vi "Untitled 3.vi"() -> ()   [LabVIEW 2020]
panel:
  out "agotado 3":string="Articulo agotado"
  in  "# dulce":dbl
  in  "#bebida fria":dbl
  in  "#cafe":dbl
  in  "# snack":dbl
  in  "stop":bool
  in  "Tab Control":enum32{"Page 1", "Page 2"}(tab)
  out "producto":bool
  out "cambio":bool
  in  "dulce":bool
  in  "bebida fria":bool
  in  "cafe":bool
  in  "snack":bool
  in  "Cancelar":bool
  in  "comprar":bool
  in  "Monedas":cluster{"moneda 10":bool, "moneda 20":bool}
  out "Cambio":dbl
  out "Dinero ingresado":dbl
  out "agotado":string="Articulo agotado"
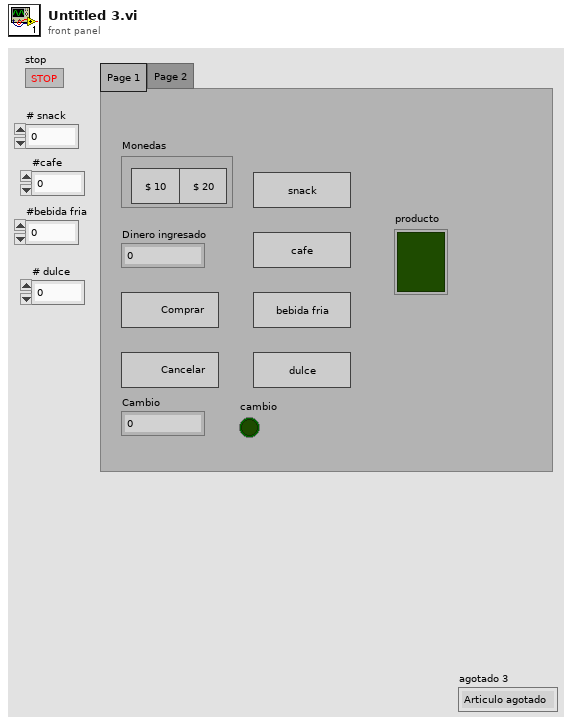
[diagram p1: front panel]
types:
  T1 = enum16{"inicio", "snack", "comprar s", "cambio s", "cafe", "comprar c", "cambio c", "bebida fria", "comprar bf", "cambio bf", "dulce", "comprar d", "cambio d", "reinicio", "cancelar"}
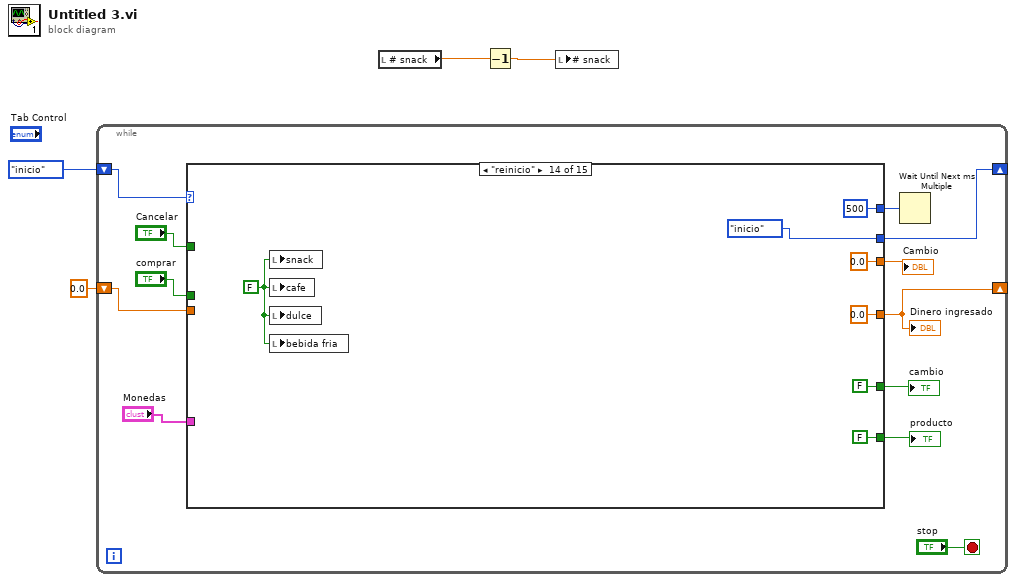
[diagram p0: block diagram]
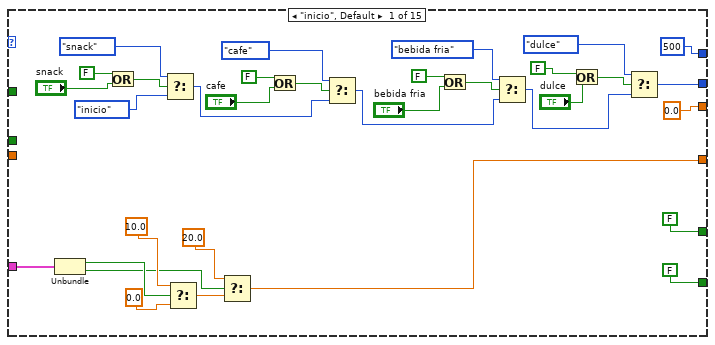
[diagram p2: hidden frame]
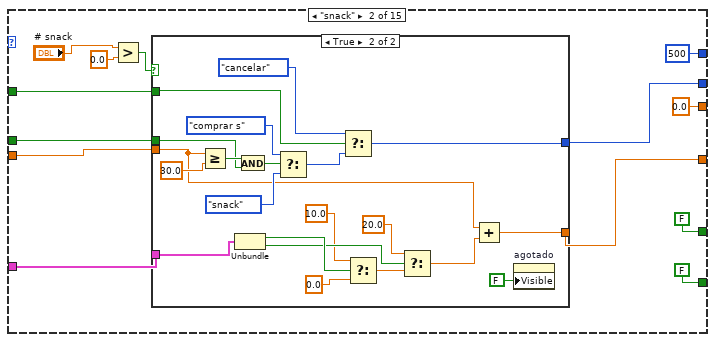
[diagram p3: hidden frame]
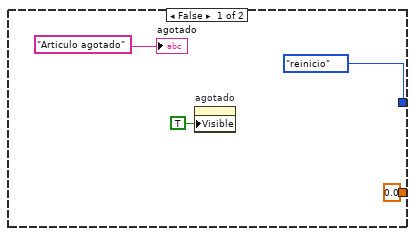
[diagram p4: hidden frame]
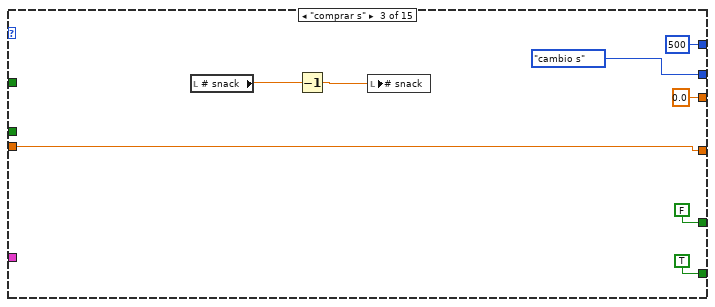
[diagram p5: hidden frame]
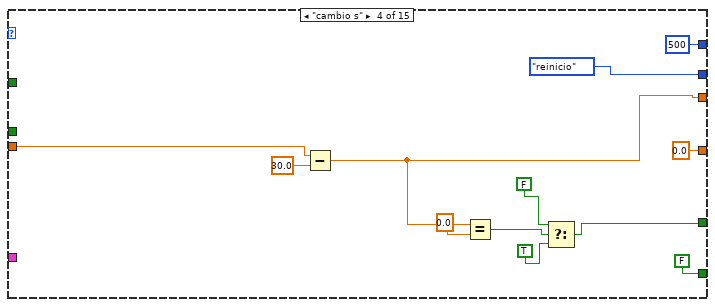
[diagram p6: hidden frame]
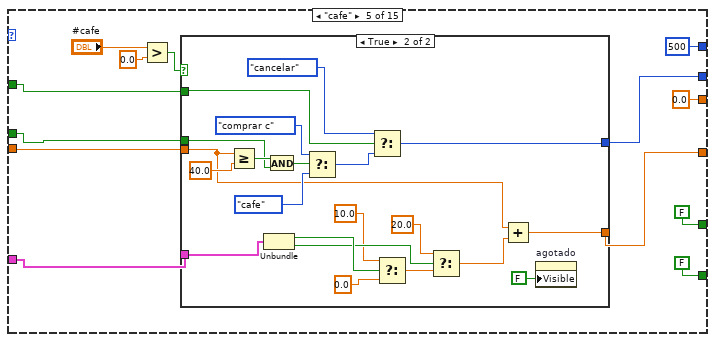
[diagram p7: hidden frame]
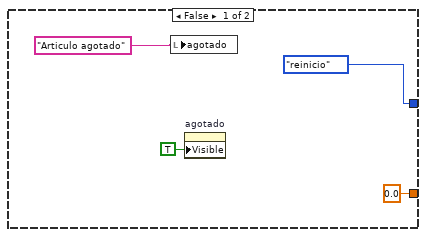
[diagram p8: hidden frame]
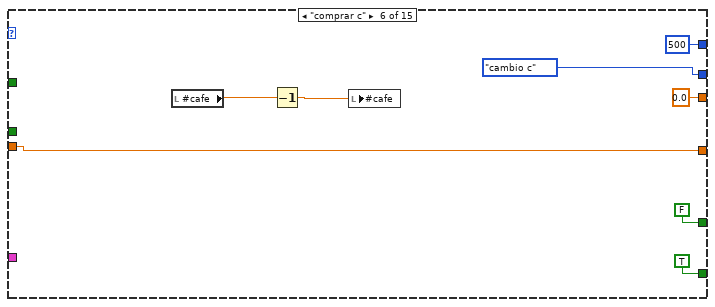
[diagram p9: hidden frame]
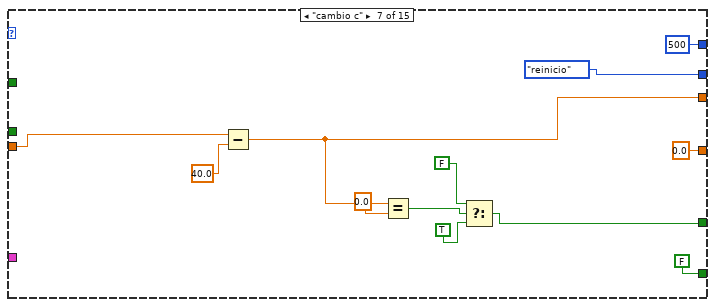
[diagram p10: hidden frame]
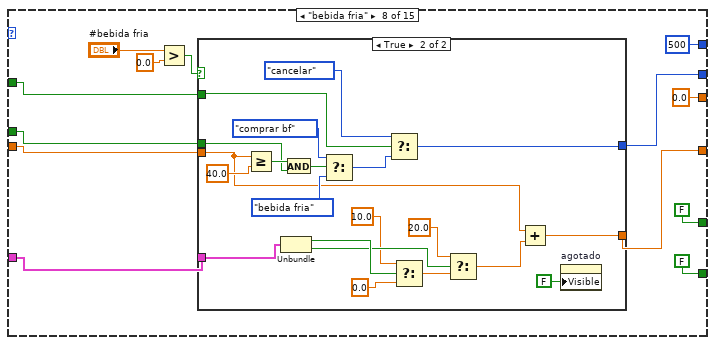
[diagram p11: hidden frame]
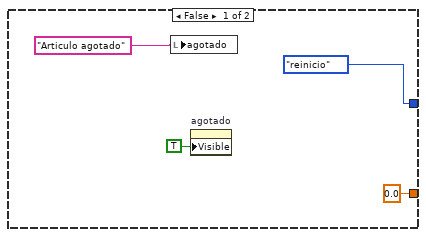
[diagram p12: hidden frame]
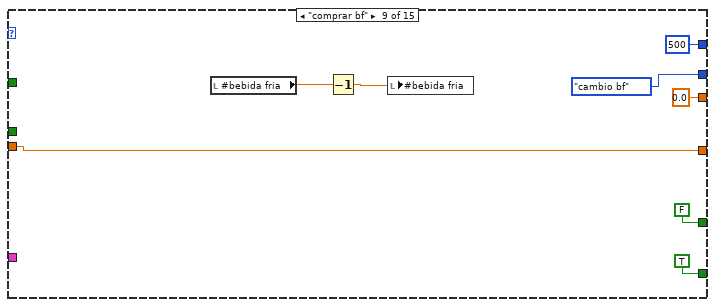
[diagram p13: hidden frame]
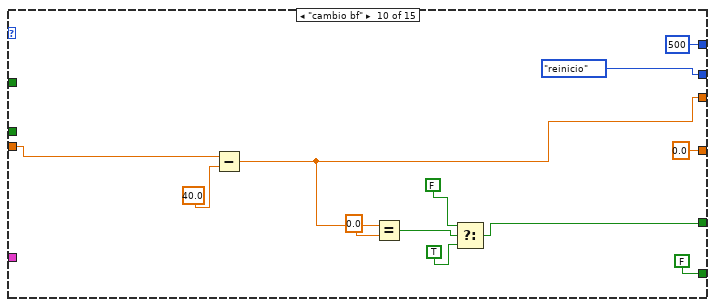
[diagram p14: hidden frame]
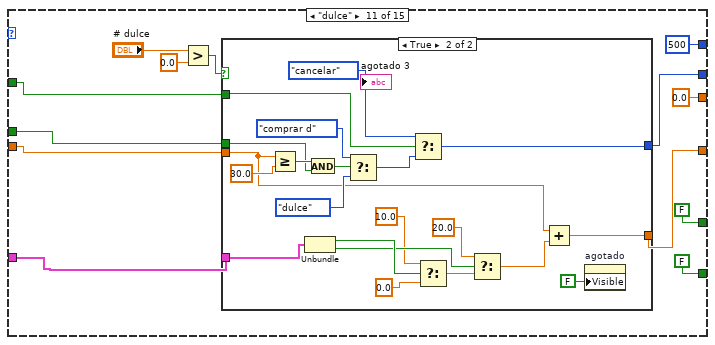
[diagram p15: hidden frame]
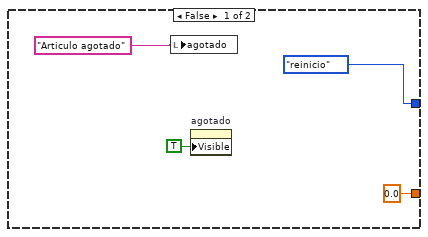
[diagram p16: hidden frame]
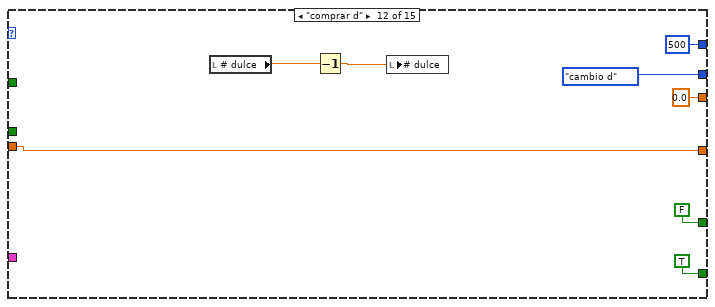
[diagram p17: hidden frame]
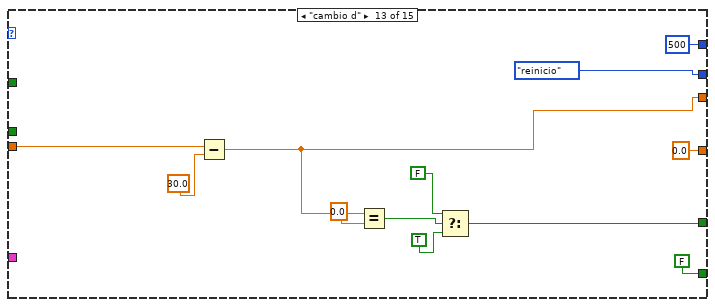
[diagram p18: hidden frame]
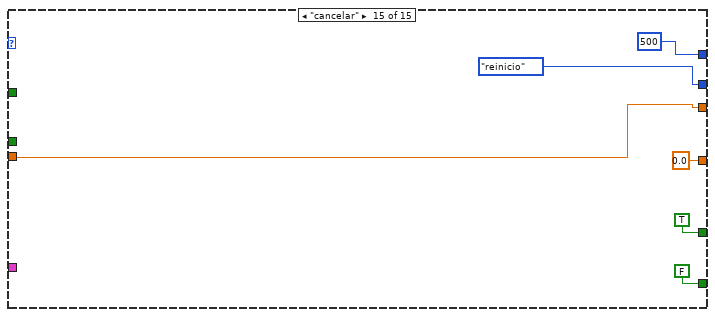
[diagram p19: hidden frame]
diagram:
  n1 = while {
    shift-right: [w14] -> _
    shift-left: T1."inicio" -> [w16]
    shift-right: [w8] -> _
    shift-left: 0.0 ("f") -> [w7]
    stop <- "stop" stop-if-true
    n2 = case shown="\"reinicio\"" w16 {
      tunnel: [500 500 500 500 500 500 500 500 500 500 500 500 500 500 500] -> w15
      tunnel: [w28 w55 T1."cambio s" T1."reinicio" w113 T1."cambio c" T1."reinicio" w171 T1."cambio bf" T1."reinicio" w228 T1."cambio d" T1."reinicio" T1."inicio" T1."reinicio"] -> w14
      tunnel: [0.0 0.0 0.0 w104 0.0 0.0 w156 0.0 0.0 w216 0.0 0.0 w273 0.0 w292] -> w13
      tunnel: "Monedas" -> [w26 w57 _ _ w114 _ _ w172 _ _ w233 _ _ _ _]
      tunnel: [w19 w56 w92 0.0 ("f") w112 w153 0.0 ("f") w168 w208 0.0 ("f") w227 w266 0.0 ("f") 0.0 ("f") 0.0 ("f")] -> w8
      tunnel: [FALSE FALSE TRUE FALSE FALSE TRUE FALSE FALSE TRUE FALSE FALSE TRUE FALSE FALSE FALSE] -> w11
      tunnel: [FALSE FALSE FALSE w100 FALSE FALSE w158 FALSE FALSE w214 FALSE FALSE w272 FALSE TRUE] -> w10
      tunnel: w7 -> [_ w60 w92 w107 w115 w153 w154 w173 w208 w212 w232 w266 w270 _ w292]
      tunnel: "comprar" -> [_ w59 _ _ w116 _ _ w174 _ _ w231 _ _ _ _]
      tunnel: "Cancelar" -> [_ w58 _ _ w117 _ _ w175 _ _ w230 _ _ _ _]
      frame "inicio", Default {
        n3 = Unbundle(w26) -> ("moneda 10"=w25:bool, "moneda 20"=w21:bool)
        n4 = Or(x=FALSE, y="snack") -> (x .or. y?=w47:bool)
        n5 = Select(t=T1."snack", s=w47, f=T1."inicio") -> (s? t:f=w40:T1)
        n6 = Select(t=10.0, s=w25, f=0.0) -> (s? t:f=w22:dbl)
        n7 = Select(t=20.0, s=w21, f=w22) -> (s? t:f=w19:dbl)
        n8 = Or(x=FALSE, y="cafe") -> (x .or. y?=w43:bool)
        n9 = Select(t=T1."cafe", s=w43, f=w40) -> (s? t:f=w35:T1)
        n10 = Or(x=FALSE, y="bebida fria") -> (x .or. y?=w38:bool)
        n11 = Select(t=T1."bebida fria", s=w38, f=w35) -> (s? t:f=w30:T1)
        n12 = Or(x=FALSE, y="dulce") -> (x .or. y?=w33:bool)
        n13 = Select(t=T1."dulce", s=w33, f=w30) -> (s? t:f=w28:T1)
      }
      frame "snack" {
        n14 = Greater?(x="# snack", y=0.0) -> (0:w61:bool)
        n15 = case shown="True" w61 {
          tunnel: w60 -> [_ w71]
          tunnel: w59 -> [_ w82]
          tunnel: w58 -> [_ w69]
          tunnel: w57 -> [_ w73]
          tunnel: [0.0 w70] -> w56
          tunnel: [T1."reinicio" w68] -> w55
          frame False {
            n16 = property on="agotado" class="Str"("Visible"=TRUE) -> ()  [unwired: 2 in, 2 out]
            "agotado" <- "Articulo agotado"
          }
          frame True {
            n17 = Greater Or Equal?(x=w71, y=30.0) -> (x >= y?=w86:bool)
            n18 = Unbundle(w73) -> ("moneda 10"=w79:bool, "moneda 20"=w77:bool)
            n19 = And(x=w86, y=w82) -> (x .and. y?=w87:bool)
            n20 = Select(t=T1."comprar s", s=w87, f=T1."snack") -> (s? t:f=w81:T1)
            n21 = Select(t=T1."cancelar", s=w69, f=w81) -> (s? t:f=w68:T1)
            n22 = Select(t=10.0, s=w79, f=0.0) -> (s? t:f=w78:dbl)
            n23 = Select(t=20.0, s=w77, f=w78) -> (s? t:f=w72:dbl)
            n24 = Add(x=w71, y=w72) -> (x+y=w70:dbl)
            n25 = property on="agotado" class="Str"("Visible"=FALSE) -> ()  [unwired: 2 in, 2 out]
          }
        }
      }
      frame "comprar s" {
        n26 = local read "# snack"() -> (w89:dbl)
        n27 = Decrement(x=w89) -> (x-1=w88:dbl)
        n28 = local write "# snack"(w88) -> ()
      }
      frame "cambio s" {
        n29 = Subtract(x=w107, y=30.0) -> (x-y=w104:dbl)
        n30 = Equal?(x=w104, y=0.0) -> (x = y?=w102:bool)
        n31 = Select(t=FALSE, s=w102, f=TRUE) -> (s? t:f=w100:bool)
      }
      frame "cafe" {
        n32 = Greater?(x="#cafe", y=0.0) -> (0:w118:bool)
        n33 = case shown="True" w118 {
          tunnel: w115 -> [_ w129]
          tunnel: w116 -> [_ w140]
          tunnel: w117 -> [_ w127]
          tunnel: w114 -> [_ w131]
          tunnel: [0.0 w128] -> w112
          tunnel: [T1."reinicio" w126] -> w113
          frame False {
            n34 = local write "agotado"("Articulo agotado") -> ()
            n35 = property on="agotado" class="Str"("Visible"=TRUE) -> ()  [unwired: 2 in, 2 out]
          }
          frame True {
            n36 = Greater Or Equal?(x=w129, y=40.0) -> (x >= y?=w144:bool)
            n37 = Unbundle(w131) -> ("moneda 10"=w137:bool, "moneda 20"=w135:bool)
            n38 = And(x=w144, y=w140) -> (x .and. y?=w145:bool)
            n39 = Select(t=T1."comprar c", s=w145, f=T1."cafe") -> (s? t:f=w139:T1)
            n40 = Select(t=T1."cancelar", s=w127, f=w139) -> (s? t:f=w126:T1)
            n41 = Select(t=10.0, s=w137, f=0.0) -> (s? t:f=w136:dbl)
            n42 = Select(t=20.0, s=w135, f=w136) -> (s? t:f=w130:dbl)
            n43 = Add(x=w129, y=w130) -> (x+y=w128:dbl)
            n44 = property on="agotado" class="Str"("Visible"=FALSE) -> ()  [unwired: 2 in, 2 out]
          }
        }
      }
      frame "comprar c" {
        n45 = local read "#cafe"() -> (w147:dbl)
        n46 = Decrement(x=w147) -> (x-1=w146:dbl)
        n47 = local write "#cafe"(w146) -> ()
      }
      frame "cambio c" {
        n48 = Subtract(x=w154, y=40.0) -> (x-y=w156:dbl)
        n49 = Equal?(x=w156, y=0.0) -> (x = y?=w161:bool)
        n50 = Select(t=FALSE, s=w161, f=TRUE) -> (s? t:f=w158:bool)
      }
      frame "bebida fria" {
        n51 = Greater?(x="#bebida fria", y=0.0) -> (0:w176:bool)
        n52 = case shown="True" w176 {
          tunnel: w173 -> [_ w187]
          tunnel: w174 -> [_ w198]
          tunnel: w175 -> [_ w185]
          tunnel: w172 -> [_ w189]
          tunnel: [0.0 w186] -> w168
          tunnel: [T1."reinicio" w184] -> w171
          frame False {
            n53 = local write "agotado"("Articulo agotado") -> ()
            n54 = property on="agotado" class="Str"("Visible"=TRUE) -> ()  [unwired: 2 in, 2 out]
          }
          frame True {
            n55 = Greater Or Equal?(x=w187, y=40.0) -> (x >= y?=w202:bool)
            n56 = Unbundle(w189) -> ("moneda 10"=w195:bool, "moneda 20"=w193:bool)
            n57 = And(x=w202, y=w198) -> (x .and. y?=w203:bool)
            n58 = Select(t=T1."comprar bf", s=w203, f=T1."bebida fria") -> (s? t:f=w197:T1)
            n59 = Select(t=T1."cancelar", s=w185, f=w197) -> (s? t:f=w184:T1)
            n60 = Select(t=10.0, s=w195, f=0.0) -> (s? t:f=w194:dbl)
            n61 = Select(t=20.0, s=w193, f=w194) -> (s? t:f=w188:dbl)
            n62 = Add(x=w187, y=w188) -> (x+y=w186:dbl)
            n63 = property on="agotado" class="Str"("Visible"=FALSE) -> ()  [unwired: 2 in, 2 out]
          }
        }
      }
      frame "comprar bf" {
        n64 = local read "#bebida fria"() -> (w205:dbl)
        n65 = Decrement(x=w205) -> (x-1=w204:dbl)
        n66 = local write "#bebida fria"(w204) -> ()
      }
      frame "cambio bf" {
        n67 = Subtract(x=w212, y=40.0) -> (x-y=w216:dbl)
        n68 = Equal?(x=w216, y=0.0) -> (x = y?=w219:bool)
        n69 = Select(t=FALSE, s=w219, f=TRUE) -> (s? t:f=w214:bool)
      }
      frame "dulce" {
        n70 = Greater?(x="# dulce", y=0.0) -> (0:w235:bool)
        n71 = case shown="True" w235 {
          tunnel: w232 -> [_ w245]
          tunnel: w231 -> [_ w256]
          tunnel: w230 -> [_ w243]
          tunnel: w233 -> [_ w247]
          tunnel: [0.0 w244] -> w227
          tunnel: [T1."reinicio" w242] -> w228
          frame False {
            n72 = local write "agotado"("Articulo agotado") -> ()
            n73 = property on="agotado" class="Str"("Visible"=TRUE) -> ()  [unwired: 2 in, 2 out]
          }
          frame True {
            n74 = Greater Or Equal?(x=w245, y=30.0) -> (x >= y?=w260:bool)
            n75 = Unbundle(w247) -> ("moneda 10"=w253:bool, "moneda 20"=w251:bool)
            n76 = And(x=w260, y=w256) -> (x .and. y?=w261:bool)
            n77 = Select(t=T1."comprar d", s=w261, f=T1."dulce") -> (s? t:f=w255:T1)
            n78 = Select(t=T1."cancelar", s=w243, f=w255) -> (s? t:f=w242:T1)
            n79 = Select(t=10.0, s=w253, f=0.0) -> (s? t:f=w252:dbl)
            n80 = Select(t=20.0, s=w251, f=w252) -> (s? t:f=w246:dbl)
            n81 = Add(x=w245, y=w246) -> (x+y=w244:dbl)
            n82 = property on="agotado" class="Str"("Visible"=FALSE) -> ()  [unwired: 2 in, 2 out]
          }
        }
      }
      frame "comprar d" {
        n83 = local read "# dulce"() -> (w263:dbl)
        n84 = Decrement(x=w263) -> (x-1=w262:dbl)
        n85 = local write "# dulce"(w262) -> ()
      }
      frame "cambio d" {
        n86 = Subtract(x=w270, y=30.0) -> (x-y=w273:dbl)
        n87 = Equal?(x=w273, y=0.0) -> (x = y?=w276:bool)
        n88 = Select(t=FALSE, s=w276, f=TRUE) -> (s? t:f=w272:bool)
      }
      frame "reinicio" {
        w282 = FALSE
        n89 = local write "snack"(w282) -> ()
        n90 = local write "cafe"(w282) -> ()
        n91 = local write "dulce"(w282) -> ()
        n92 = local write "bebida fria"(w282) -> ()
      }
      frame "cancelar" {
      }
    }
    "Cambio" <- w13
    "Dinero ingresado" <- w8
    "cambio" <- w10
    "producto" <- w11
    n93 = Wait Until Next ms Multiple(millisecond multiple=w15) -> ()  [unwired: 1 out]
  }
  n94 = local read "# snack"() -> (w1:dbl)
  n95 = Decrement(x=w1) -> (x-1=w2:dbl)
  n96 = local write "# snack"(w2) -> ()
